vi "Dispose Test Object.vi"(8 "error in (no error)":errorcluster, 11 "Numeric":refnum<class "Numeric Test Object.lvclass">) -> (0 "error out":errorcluster)   [LabVIEW 2009]
doc: "Disposes of all references used by the numeric test object."
uses:
  Numeric Test Object/Numeric Test Object.lvclass
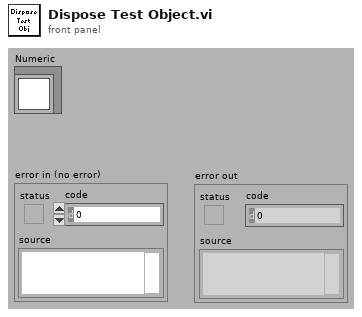
[diagram p1: front panel]
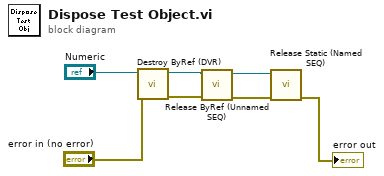
[diagram p0: block diagram]
diagram:
  n1 = call-dynamic "Destroy ByRef (DVR).vi"("error in (no error)"="error in (no error)", "Numeric in"="Numeric") -> ("error out"=w3:errorcluster, "Numeric out"=w6:refnum<class "Numeric Test Object.lvclass">)  [unwired: 8 in]
  n2 = call-dynamic "Release ByRef (Unnamed SEQ).vi"("error in (no error)"=w3, "Numeric in"=w6) -> ("error out"=w2:errorcluster, "Numeric out"=w5:refnum<class "Numeric Test Object.lvclass">)  [unwired: 8 in]
  n3 = call-dynamic "Release Static (Named SEQ).vi"("error in (no error)"=w2, "Numeric in"=w5) -> ("error out"=→"error out":errorcluster)  [unwired: 8 in, 1 out]
